vi "ultrasonic.vi"() -> ()   [LabVIEW 2022 SP3]
uses:
  <vilib>/DAQmx/read.llb/DAQmx Read (Analog Wfm 1Chan NSamp).vi
  <vilib>/DAQmx/write.llb/DAQmx Write (Digital Bool 1Line 1Point).vi
  <vilib>/DAQmx/create/channels.llb/DAQmx Create Channel (DO-Digital Output).vi
  <vilib>/DAQmx/miscellaneous.llb/DAQmx Fill In Error Info.vi
  <vilib>/DAQmx/create/channels.llb/DAQmx Create Channel (AI-Voltage-Basic).vi
  <vilib>/DAQmx/configure/timing.llb/DAQmx Timing (Sample Clock).vi
panel:
  out "Distance":dbl format="%#_3g"
  out "Waveform Graph":waveform(dbl)(graph)
  in  "DAQmx Physical Channel 2":tag
  in  "DAQmx Physical Channel":tag
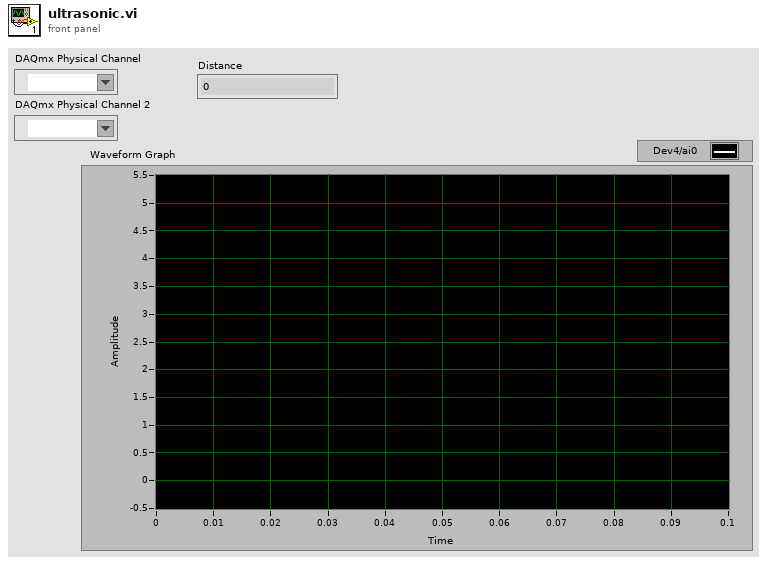
[diagram p1: front panel]
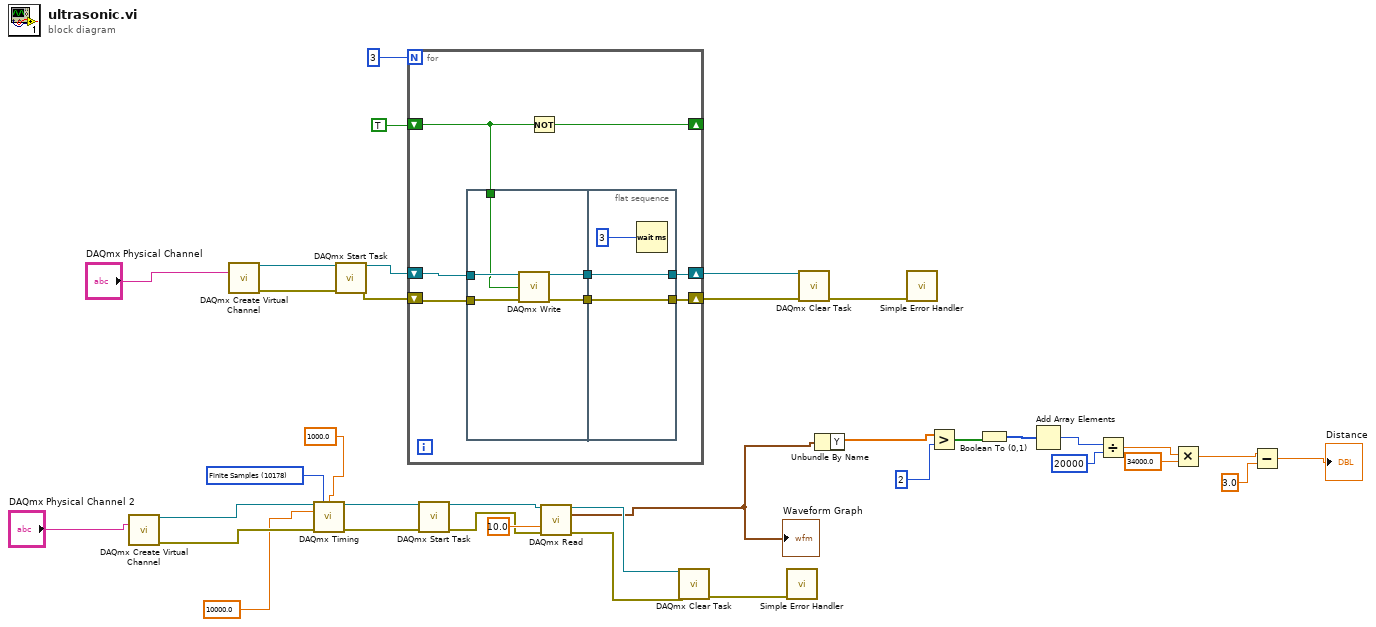
[diagram p0: block diagram]
diagram:
  w25 = 10178 items=["Finite Samples"=10178, "Continuous Samples"=10123, "Hardware Timed Single Point"=12522] ("sample mode")
  n1 = call-poly <vilib>:"DAQmx Create Virtual Channel.vi"("physical channels"="DAQmx Physical Channel 2") -> ("task out"=w24:refnum<k21>, "error out"=w23:errorcluster)  [unwired: 13 in]
  n2 = call-poly <vilib>:"DAQmx Create Virtual Channel.vi"("lines"="DAQmx Physical Channel") -> ("task out"=w35:refnum<k21>, "error out"=w34:errorcluster)  [unwired: 13 in]
  n3 = call-poly <vilib>:"DAQmx Timing.vi"("task/channels in"=w24, "sample mode"=w25, "samples per channel"=1000.0 ("Number of samples"), "rate"=10000.0 ("Sampling frequency"), "error in"=w23) -> ("task out"=w22:refnum<k21>, "error out"=w21:errorcluster)  [unwired: 9 in]
  n4 = call <vilib>:"DAQmx Start Task.vi"("task/channels in"=w35, "error in"=w34) -> ("task out"=w33:refnum<k21>, "error out"=w32:errorcluster)  [unwired: 12 in]
  n5 = for {
    N: 3 -> [_]
    shift-right: [w40] -> w30
    shift-left: w33 -> [w42]
    shift-right: [w39] -> w29
    shift-left: w32 -> [w41]
    shift-right: [w38] -> _
    shift-left: TRUE -> [w37]
    n6 = flat-sequence {
      tunnel: w42 -> [w49]
      tunnel: w41 -> [w48]
      tunnel: [w47] -> w44
      tunnel: [w46] -> w43
      tunnel: w37 -> [w45]
      tunnel: [w51] -> w40
      tunnel: w44 -> [w51]
      tunnel: [w50] -> w39
      tunnel: w43 -> [w50]
      frame #0 {
        n7 = call-poly <vilib>:"DAQmx Write.vi"("task/channels in"=w49, "data"=w45, "error in"=w48) -> ("task out"=w47:refnum<k21>, "error out"=w46:errorcluster)  [unwired: 10 in, 1 out]
      }
      frame #1 {
        n8 = Wait (ms)(milliseconds to wait=u32 3) -> ()  [unwired: 1 out]
      }
    }
    n9 = Not(x=w37) -> (.not. x?=w38:bool)
  }
  n10 = call <vilib>:"DAQmx Start Task.vi"("task/channels in"=w22, "error in"=w21) -> ("task out"=w19:refnum<k21>, "error out"=w18:errorcluster)  [unwired: 12 in]
  n11 = call-poly <vilib>:"DAQmx Read.vi"("task/channels in"=w19, "timeout"=10.0, "error in"=w18) -> ("task out"=w13:refnum<k21>, "data"=w10:waveform(dbl), "error out"=w16:errorcluster)  [unwired: 10 in]
  "Waveform Graph" <- w10
  n12 = call <vilib>:"DAQmx Clear Task.vi"("task in"=w13, "error in"=w16) -> ("error out"=w17:errorcluster)  [unwired: 13 in]
  n13 = call <vilib>:"Simple Error Handler.vi"("error in (no error)"=w17) -> ()  [unwired: 4 in, 5 out]
  n14 = call <vilib>:"DAQmx Clear Task.vi"("task in"=w30, "error in"=w29) -> ("error out"=w31:errorcluster)  [unwired: 13 in]
  n15 = Unbundle By Name(w10) -> ("Y"=w11:dbl[])
  n16 = call <vilib>:"Simple Error Handler.vi"("error in (no error)"=w31) -> ()  [unwired: 4 in, 5 out]
  n17 = Greater?(x=w11, y=2) -> (0:w9:bool[])
  n18 = Boolean To (0,1)(Boolean=w9) -> (0, 1=w8:i16[])
  n19 = Add Array Elements(numeric array=w8) -> (sum=w4:i16)
  n20 = Divide(x=w4, y=i16 20000) -> (x/y=w5:dbl)
  n21 = Multiply(x=w5, y=34000.0) -> (x*y=w3:dbl)
  n22 = Subtract(x=w3, y=3.0) -> (x-y=→"Distance":dbl)
